vi "Exponential - RM.vi"(1 "Real Matrix A":T1) -> (0 "e^A":T1)   [LabVIEW 2020, in "NI_Matrix.lvlib"]
doc: "Computes the exponential of the input matrix."
uses:
  NI_Matrix.lvlib
  RealMatrix.ctl
  Real Matrix Exp.vi
  NI_AALBase.lvlib
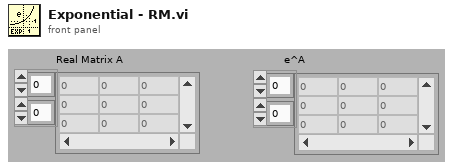
[diagram p1: front panel]
types:
  T1 = typedef "NI_Matrix.lvlib/RealMatrix.ctl" = dbl[][]
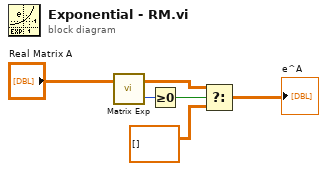
[diagram p0: block diagram]
diagram:
  n1 = call-poly "Matrix Exp.vi"("Input Matrix"="Real Matrix A") -> ("error"=w1:i32, "Matrix Exp"=w2:T1)  [unwired: 1 in]
  n2 = Greater Or Equal To 0?(x=w1) -> (x >= 0?=w6:bool)
  n3 = Select(t=w2, s=w6, f=T1 [] ("sqrt(A)")) -> (s? t:f=→"e^A":T1)
